vi "main.vi"() -> ()   [LabVIEW 2015]
uses:
  <vilib>/myRIO/Instrument Drivers/Onboard IO/DIO/typedefs/DIO Reference.ctl
  <vilib>/myRIO/Common/Instrument Driver Framework/Utilities/typedefs/myRIO Generic Hardware Reference.ctl
  <vilib>/myRIO/Common/Instrument Driver Framework/Utilities/typedefs/Hardware Version Enum.ctl
  <vilib>/myRIO/Common/Instrument Driver Framework/Utilities/typedefs/myRIO v1.0 Reference.ctl
  <vilib>/myRIO/Common/Instrument Driver Framework/Utilities/typedefs/Generic FPGA Reference.ctl
  <vilib>/myRIO/Common/Instrument Driver Framework/myRIO v1.0/DIO/typedefs/DIO Channels List.ctl
  <vilib>/myRIO/Common/Instrument Driver Framework/myRIO v1.0/DIO/typedefs/DIO Channels Enum.ctl
  <vilib>/userdefined/High Color/nirio_resource_hc.ctl
  <vilib>/myRIO/Instrument Drivers/Onboard IO/AO/typedefs/AO Reference.ctl
  <vilib>/myRIO/Common/Instrument Driver Framework/myRIO v1.0/AO/typedefs/AO Channels List.ctl
  <vilib>/myRIO/Common/Instrument Driver Framework/myRIO v1.0/AO/typedefs/AO Channels Enum.ctl
  <vilib>/myRIO/Common/Instrument Driver Framework/Utilities/typedefs/Analog Scaling Constants List.ctl
  <vilib>/myRIO/Common/Instrument Driver Framework/Utilities/typedefs/Analog Scaling Constants.ctl
  <vilib>/myRIO/Instrument Drivers/Onboard IO/SPI/typedefs/SPI User Configuration.ctl
  <vilib>/myRIO/Common/Instrument Driver Framework/myRIO v1.0/SPI/typedefs/SPI Clock Phase.ctl
  <vilib>/myRIO/Common/Instrument Driver Framework/myRIO v1.0/SPI/typedefs/SPI Clock Polarity.ctl
  <vilib>/myRIO/Common/Instrument Driver Framework/myRIO v1.0/SPI/typedefs/SPI Data Direction.ctl
  <vilib>/myRIO/Common/Instrument Driver Framework/myRIO v1.0/SPI/typedefs/SPI Frame Length.ctl
  <vilib>/myRIO/Instrument Drivers/Onboard IO/SPI/typedefs/SPI Reference.ctl
  <vilib>/myRIO/Common/Instrument Driver Framework/myRIO v1.0/SPI/typedefs/SPI Channels Enum.ctl
  <vilib>/myRIO/Instrument Drivers/Onboard IO/SPI/typedefs/SPI Configuration.ctl
  <vilib>/myRIO/Common/Instrument Driver Framework/Utilities/vis/Is FPGA Ref Available.vi
  <vilib>/myRIO/Common/Instrument Driver Framework/myRIO v1.0/DIO/vis/myRIO v1.1 Open DIO.vi
  <vilib>/myRIO/Instrument Drivers/Onboard IO/DIO/vis/Write.vi
  <vilib>/myRIO/Common/Instrument Driver Framework/myRIO v1.0/AO/vis/myRIO v1.1 Open AO.vi
  <vilib>/myRIO/Instrument Drivers/Onboard IO/AO/vis/Write.vi
  <vilib>/myRIO/Common/Instrument Driver Framework/myRIO v1.0/SPI/vis/myRIO v1.1 Open SPI.vi
  <vilib>/myRIO/Instrument Drivers/Onboard IO/SPI/vis/Configure.vi
  <vilib>/myRIO/Instrument Drivers/Onboard IO/SPI/vis/Write Read.vi
  <vilib>/myRIO/Common/Instrument Driver Framework/Utilities/vis/Validate Channels.vi
  <vilib>/myRIO/Common/Instrument Driver Framework/myRIO v1.0/DIO/vis/myRIO v1.0 Reserve DIO.vi
  <vilib>/myRIO/Common/Instrument Driver Framework/myRIO v1.0/AO/vis/myRIO v1.0 Reserve AO.vi
  <vilib>/myRIO/Common/Instrument Driver Framework/myRIO v1.0/SPI/vis/myRIO v1.0 Reserve SPI.vi
  <vilib>/myRIO/Common/Instrument Driver Framework/myRIO v1.0/Resource Manager/vis/myRIO v1.0 Reserve Channel List.vi
  <vilib>/myRIO/Common/Instrument Driver Framework/myRIO v1.0/DIO/vis/myRIO v1.0 Build MUX Configuration DIO.vi
  <vilib>/myRIO/Common/Instrument Driver Framework/myRIO v1.0/AO/vis/myRIO v1.0 Build MUX Configuration AO.vi
  <vilib>/myRIO/Common/Instrument Driver Framework/myRIO v1.0/SPI/vis/myRIO v1.0 Build MUX Configuration SPI.vi
  <vilib>/myRIO/Common/Instrument Driver Framework/myRIO v1.0/Resource Manager/vis/myRIO v1.0 Reserve Channel.vi
  <vilib>/myRIO/Common/Instrument Driver Framework/myRIO v1.0/Resource Manager/vis/myRIO v1.0 Unreserve Channel.vi
  <vilib>/myRIO/Common/Instrument Driver Framework/myRIO v1.0/Resource Manager/vis/myRIO v1.0 Create Configuration List.vi
  <vilib>/myRIO/Common/Instrument Driver Framework/myRIO v1.0/Resource Manager/vis/myRIO v1.0 Build Mutex Name.vi
  <vilib>/Utility/VariantDataType/GetNumericInfo.vi
  <vilib>/Utility/error.llb/Error Cluster From Error Code.vi
  <vilib>/myRIO/Common/Instrument Driver Framework/myRIO v1.0/myRIO v1.1 Open.vi
  <vilib>/myRIO/Common/Instrument Driver Framework/Utilities/vis/IO Manager.vi
  <vilib>/myRIO/Common/Instrument Driver Framework/Utilities/vis/Configuration Manager.vi
  <vilib>/myRIO/Common/Instrument Driver Framework/myRIO v1.0/Resource Manager/vis/myRIO v1.0 Configure IO.vi
  <vilib>/myRIO/Common/Instrument Driver Framework/myRIO v1.0/myRIO v1.0 Close.vi
  <vilib>/myRIO/Common/Instrument Driver Framework/myRIO v1.0/DIO/vis/myRIO v1.0 Write DIO.vi
  <vilib>/myRIO/Common/Instrument Driver Framework/myRIO v1.0/SPI/vis/myRIO v1.0 Configure SPI.vi
  <vilib>/myRIO/Common/Instrument Driver Framework/myRIO v1.0/SPI/vis/myRIO v1.0 Write Read SPI.vi
  <vilib>/myRIO/Common/Instrument Driver Framework/myRIO v1.0/AO/vis/myRIO v1.0 Get Scaling Constants AO.vi
  <vilib>/myRIO/Common/Instrument Driver Framework/myRIO v1.0/AO/vis/myRIO v1.0 Write AO.vi
  <vilib>/myRIO/Express VI/Onboard IO/DO/DO Express VI.xnode
  <vilib>/myRIO/Instrument Drivers/Onboard IO/DIO/vis/myRIO DIO Open.xnode
  <vilib>/myRIO/Express VI/Onboard IO/SPI/SPI Express VI.xnode
  <vilib>/myRIO/Instrument Drivers/Onboard IO/SPI/vis/myRIO SPI Open.xnode
  <vilib>/myRIO/Express VI/Onboard IO/AO/AO Express VI.xnode
  <vilib>/myRIO/Instrument Drivers/Onboard IO/AO/vis/myRIO AO Open.xnode
  <vilib>/myRIO/Instrument Drivers/Onboard IO/DIO/DIO.lvlib
  <vilib>/myRIO/Instrument Drivers/Onboard IO/SPI/SPI.lvlib
  <vilib>/myRIO/Instrument Drivers/Onboard IO/AO/AO.lvlib
panel:
  in  "Speed":dbl(slide) scale=0.0..2.0
  in  "Maximum Limitation/degree":dbl
  in  "Minimum Limitation/degree":dbl
  out "speed in mode 1":dbl
  in  "Pattern":string(combo)
  out "Real-time Angle":dbl
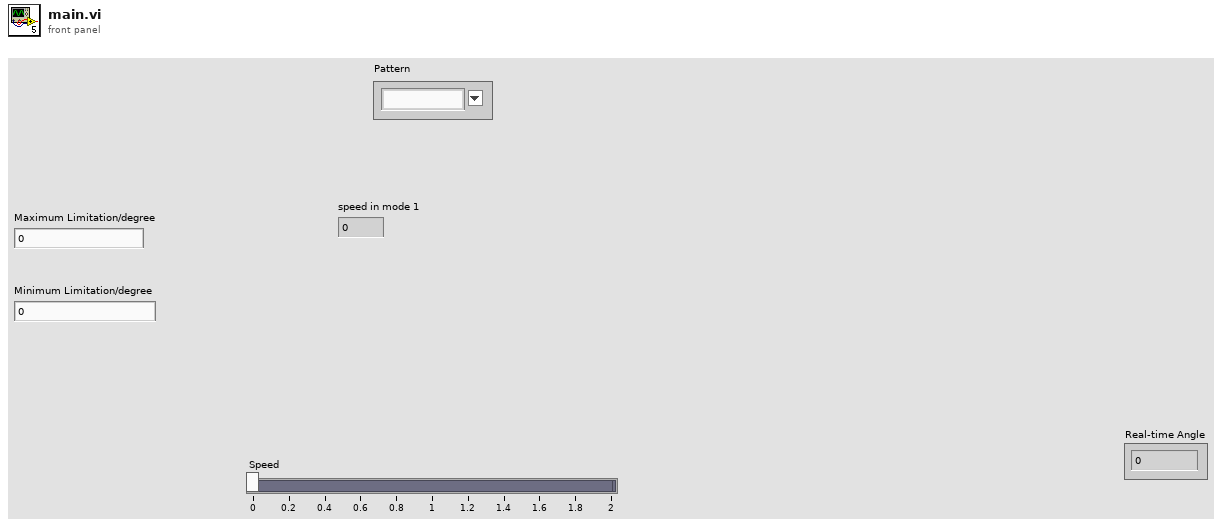
[diagram p1: front panel]
types:
  T1 = typedef "DIO.lvlib/DIO Reference.ctl" = cluster{"myRIO Reference":T2, "DIO Channels List":T6}
  T2 = typedef "myRIO Generic Hardware Reference.ctl" = cluster{"myRIO Model":T3, "myRIO Hardware Reference":T4}
  T3 = typedef "Hardware Version Enum.ctl" = enum16{"Unknown", "myRIO-1900", "myRIO-1950", "roboRIO"}
  T4 = typedef "myRIO v1.0 Reference.ctl" = cluster{"Generic FPGA Reference":T5, "Allow multiple opens":bool}
  T5 = typedef "Generic FPGA Reference.ctl" = refnum<k20>
  T6 = typedef "DIO Channels List.ctl" = T7[]
  T7 = typedef "DIO Channels Enum.ctl" = enum16{"Not Connected", "C/DIO0", "C/DIO1", "C/DIO2", "C/DIO3", "C/DIO4", "C/DIO5", "C/DIO6", "C/DIO7", "A/DIO0", "A/DIO1", "A/DIO2", "A/DIO3", "A/DIO4", "A/DIO5", "A/DIO6", "A/DIO7", "A/DIO8", "A/DIO9", "A/DIO10", "A/DIO11", "A/DIO12", "A/DIO13", "A/DIO14", "A/DIO15", "B/DIO0", "B/DIO1", "B/DIO2", "B/DIO3", "B/DIO4", "B/DIO5", "B/DIO6", "B/DIO7", "B/DIO8", "B/DIO9", "B/DIO10", "B/DIO11", "B/DIO12", "B/DIO13", "B/DIO14", "B/DIO15", "LED0", "LED1", "LED2", "LED3", "Button0", "DIO/DIO0", "DIO/DIO1", "DIO/DIO2", "DIO/DIO3", "DIO/DIO4", "DIO/DIO5", "DIO/DIO6", "DIO/DIO7", "DIO/DIO8", "DIO/DIO9", "SPI/CS0", "SPI/CS1", "SPI/CS2", "SPI/CS3", "LED RADIO (Green)", "LED RADIO (Red)", "LED COMM (Green)", "LED COMM (Red)", "LED MODE (Green)", "LED MODE (Red)"}
  T8 = typedef "nirio_resource_hc.ctl" = tag
  T9 = typedef "SPI.lvlib/SPI Reference.ctl" = cluster{"myRIO Reference":T2, "SPI Channels Enum":T10, "SPI Configuration":T11}
  T10 = typedef "SPI Channels Enum.ctl" = enum16{"Not Connected", "A/SPI", "B/SPI", "SPI/SPI"}
  T11 = typedef "SPI.lvlib/SPI Configuration.ctl" = cluster{"Frequency [Hz]":dbl, "Clock Phase":T12, "Clock Polarity":T13, "Data Direction":T14, "Frame Length":T15}
  T12 = typedef "SPI Clock Phase.ctl" = enum8{"Leading", "Trailing"}
  T13 = typedef "SPI Clock Polarity.ctl" = enum8{"Low", "High"}
  T14 = typedef "SPI Data Direction.ctl" = enum8{"Most significant bit first", "Least significant bit first"}
  T15 = typedef "SPI Frame Length.ctl" = u8
  T16 = typedef "SPI.lvlib/SPI User Configuration.ctl" = cluster{"Frequency [Hz]":dbl, "Clock Phase":T12, "Clock Polarity":T13, "Data Direction":T14, "Frame Length":T15}
  T17 = typedef "AO.lvlib/AO Reference.ctl" = cluster{"myRIO Reference":T2, "AO Channel List":T18, "AO Scaling Constant List":T20}
  T18 = typedef "AO Channels List.ctl" = T19[]
  T19 = typedef "AO Channels Enum.ctl" = enum16{"Not Connected", "AudioOut/Left", "AudioOut/Right", "C/AO0", "C/AO1", "A/AO0", "A/AO1", "B/AO0", "B/AO1"}
  T20 = typedef "Analog Scaling Constants List.ctl" = T21[]
  T21 = typedef "Analog Scaling Constants.ctl" = cluster{"LSB Weight (Volts)":dbl, "Offset (Volts)":dbl, "Signed?":bool}
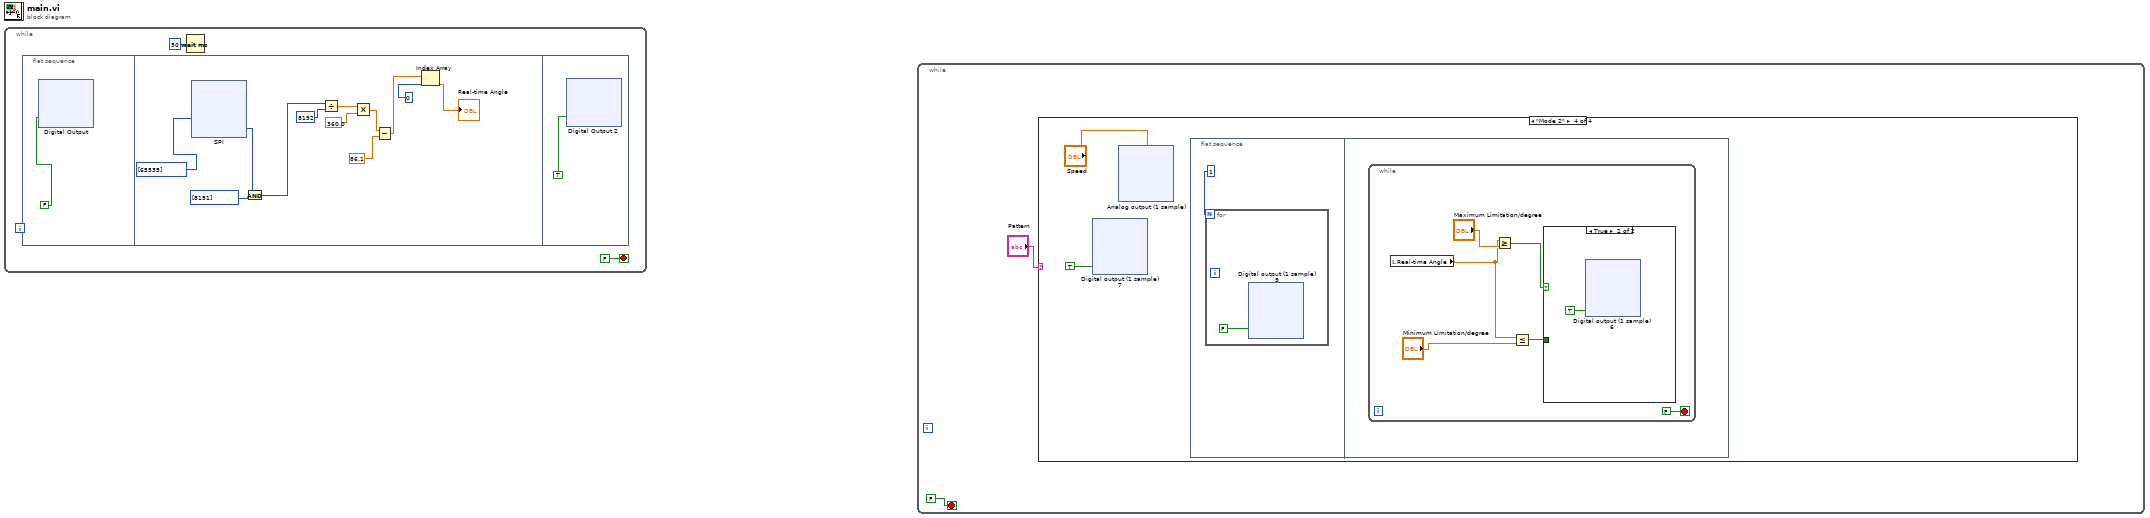
[diagram p0: block diagram]
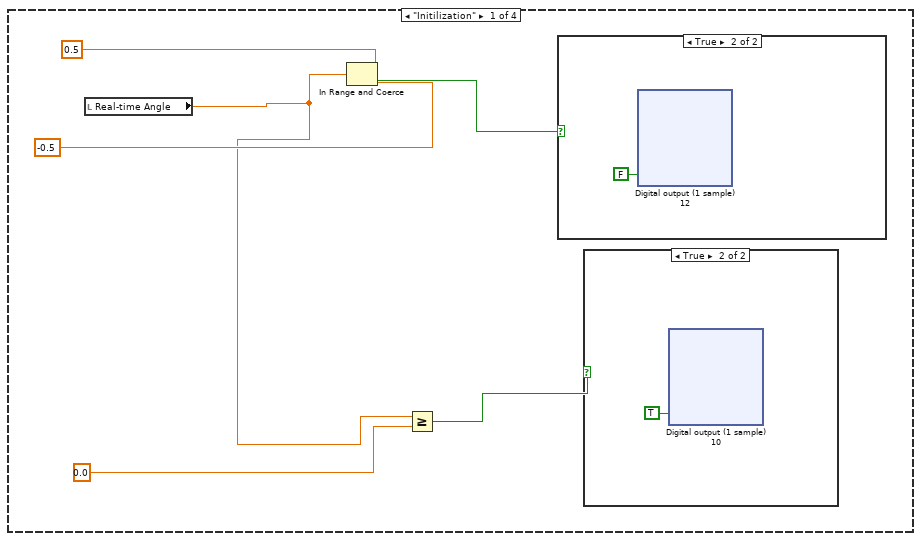
[diagram p2: hidden frame]
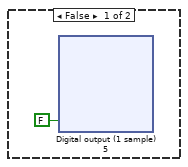
[diagram p3: hidden frame]
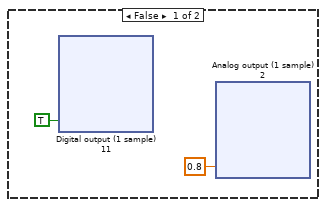
[diagram p4: hidden frame]
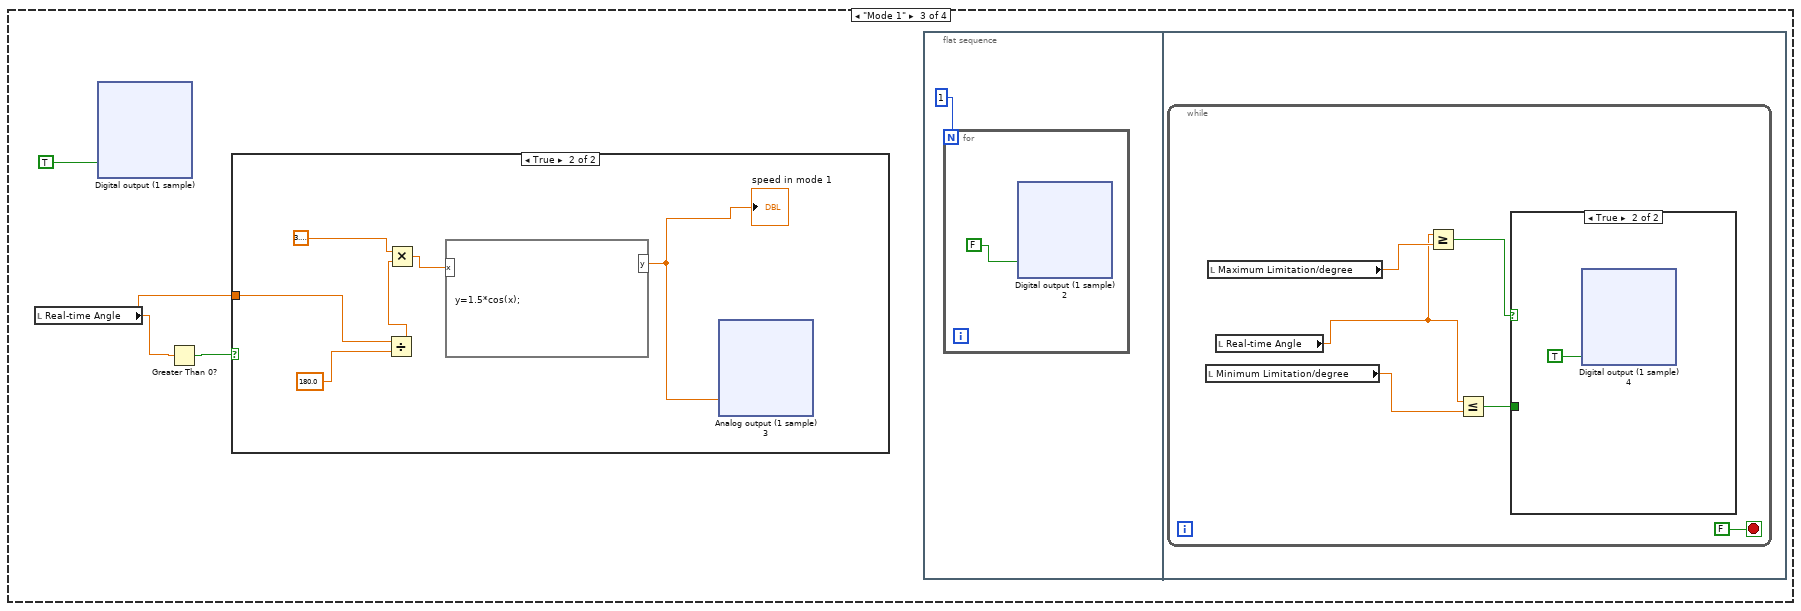
[diagram p6: hidden frame]
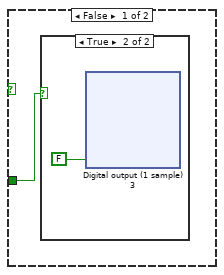
[diagram p7: hidden frame]
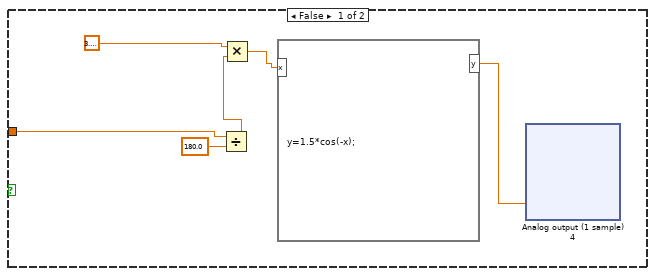
[diagram p9: hidden frame]
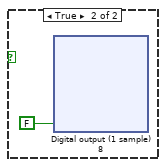
[diagram p11: hidden frame]
diagram:
  n1 = while {
    stop <- FALSE stop-if-true
    n2 = flat-sequence {
      frame #0 {
        n3 = xnode "Digital Output"("B/DIO15 (Pin 34)"=FALSE ("B/DIO0 (Pin 11)")) -> ()  [unwired: 1 in, 1 out]
      }
      frame #1 {
        n4 = xnode "SPI"("Frames to Write"=u16[] [65535]) -> ("Frames Read"=w44:u16[])  [unwired: 1 in, 1 out]
        n5 = And(x=w44, y=u16[] [8191]) -> (x .and. y?=w43:u16[])
        n6 = Divide(x=w43, y=u16 8192) -> (x/y=w45:dbl[])
        n7 = Multiply(x=w45, y=360.0) -> (x*y=w41:dbl[])
        n8 = Subtract(x=w41, y=86.1) -> (x-y=w40:dbl[])
        n9 = Index Array(array=w40, index=0) -> (element=→"Real-time Angle":dbl)
      }
      frame #2 {
        n10 = xnode "Digital Output 2"("B/DIO15 (Pin 34)"=TRUE ("B/DIO0 (Pin 11)")) -> ()  [unwired: 1 in, 1 out]
      }
    }
    n11 = Wait (ms)(milliseconds to wait=u32 50) -> ()  [unwired: 1 out]
  }
  n12 = while {
    stop <- FALSE stop-if-true
    n13 = case shown="\"Mode 2\"" "Pattern" {
      frame "Initilization" {
        n14 = local read "Real-time Angle"() -> (w127:dbl)
        n15 = In Range and Coerce(upper limit=0.5, x=w127, lower limit=-0.5) -> (In Range?=w128:bool)  [unwired: 1 out]
        n16 = Greater Or Equal?(x=w127, y=0.0) -> (x >= y?=w131:bool)
        n17 = case shown="True" w128 {
          frame False {
            n18 = xnode "Digital output (1 sample) 11"("A/DIO2 (Pin 15)"=TRUE) -> ()  [unwired: 1 in, 1 out]
            n19 = xnode "Analog output (1 sample) 2"("A/AO1 (Pin 4)"=0.8) -> ()  [unwired: 1 in, 1 out]
          }
          frame True {
            n20 = xnode "Digital output (1 sample) 12"("A/DIO2 (Pin 15)"=FALSE) -> ()  [unwired: 1 in, 1 out]
          }
        }
        n21 = case shown="True" w131 {
          frame False {
            n22 = xnode "Digital output (1 sample) 5"("A/DIO3 (Pin 17)"=FALSE) -> ()  [unwired: 1 in, 1 out]
          }
          frame True {
            n23 = xnode "Digital output (1 sample) 10"("A/DIO3 (Pin 17)"=TRUE) -> ()  [unwired: 1 in, 1 out]
          }
        }
      }
      frame Default {
      }
      frame "Mode 1" {
        n24 = local read "Real-time Angle"() -> (w315:dbl)
        n25 = xnode "Digital output (1 sample)"("A/DIO2 (Pin 15)"=TRUE) -> ()  [unwired: 1 in, 1 out]
        n26 = Greater Than 0?(x=w315) -> (x > 0?=w316:bool)
        n27 = case shown="True" w316 {
          tunnel: w315 -> [w434 w478]
          frame False {
            n28 = Divide(x=w434, y=180.0) -> (x/y=w439:dbl)
            n29 = Multiply(x=3.141592653589793, y=w439) -> (x*y=w438:dbl)
            n30 = formula code="y=1.5*cos(-x);"("x"=w438) -> ("y"=w435:dbl)
            n31 = xnode "Analog output (1 sample) 4"("A/AO1 (Pin 4)"=w435) -> ()  [unwired: 1 in, 1 out]
          }
          frame True {
            n32 = Divide(x=w478, y=180.0 ("x")) -> (x/y=w482:dbl)
            n33 = Multiply(x=3.141592653589793, y=w482) -> (x*y=w481:dbl)
            n34 = formula code="y=1.5*cos(x);"("x"=w481) -> ("y"=w477:dbl)
            "speed in mode 1" <- w477
            n35 = xnode "Analog output (1 sample) 3"("A/AO1 (Pin 4)"=w477) -> ()  [unwired: 1 in, 1 out]
          }
        }
        n36 = flat-sequence {
          frame #0 {
            n37 = for {
              N: 1 -> [_]
              n38 = xnode "Digital output (1 sample) 2"("A/DIO3 (Pin 17)"=FALSE) -> ()  [unwired: 1 in, 1 out]
            }
          }
          frame #1 {
            n39 = while {
              stop <- FALSE stop-if-true
              n40 = local read "Minimum Limitation/degree"() -> (w356:dbl)
              n41 = local read "Maximum Limitation/degree"() -> (w357:dbl)
              n42 = local read "Real-time Angle"() -> (w355:dbl)
              n43 = Greater Or Equal?(x=w355, y=w357) -> (x >= y?=w360:bool)
              n44 = Less Or Equal?(x=w355, y=w356) -> (x <= y?=w359:bool)
              n45 = case shown="True" w360 {
                tunnel: w359 -> [w361 _]
                frame False {
                  n46 = case shown="True" w361 {
                    frame False {
                    }
                    frame True {
                      n47 = xnode "Digital output (1 sample) 3"("A/DIO3 (Pin 17)"=FALSE) -> ()  [unwired: 1 in, 1 out]
                    }
                  }
                }
                frame True {
                  n48 = xnode "Digital output (1 sample) 4"("A/DIO3 (Pin 17)"=TRUE) -> ()  [unwired: 1 in, 1 out]
                }
              }
            }
          }
        }
      }
      frame "Mode 2" {
        n49 = xnode "Digital output (1 sample) 7"("A/DIO2 (Pin 15)"=TRUE) -> ()  [unwired: 1 in, 1 out]
        n50 = xnode "Analog output (1 sample)"("A/AO1 (Pin 4)"="Speed") -> ()  [unwired: 1 in, 1 out]
        n51 = flat-sequence {
          frame #0 {
            n52 = for {
              N: 1 -> [_]
              n53 = xnode "Digital output (1 sample) 9"("A/DIO3 (Pin 17)"=FALSE) -> ()  [unwired: 1 in, 1 out]
            }
          }
          frame #1 {
            n54 = while {
              stop <- FALSE stop-if-true
              n55 = local read "Real-time Angle"() -> (w629:dbl)
              n56 = Greater Or Equal?(x=w629, y="Maximum Limitation/degree") -> (x >= y?=w633:bool)
              n57 = Less Or Equal?(x=w629, y="Minimum Limitation/degree") -> (x <= y?=w632:bool)
              n58 = case shown="True" w633 {
                tunnel: w632 -> [w635 _]
                frame False {
                  n59 = case shown="False" w635 {
                    frame False {
                    }
                    frame True {
                      n60 = xnode "Digital output (1 sample) 8"("A/DIO3 (Pin 17)"=FALSE) -> ()  [unwired: 1 in, 1 out]
                    }
                  }
                }
                frame True {
                  n61 = xnode "Digital output (1 sample) 6"("A/DIO3 (Pin 17)"=TRUE) -> ()  [unwired: 1 in, 1 out]
                }
              }
            }
          }
        }
      }
    }
  }
